vi "ADO Connection Create Table if Not Exist.vi"(6 "use file? (F)":bool, 7 "parameters":T1[](array[typedef]), 8 "error in (no error)":errorcluster caption="错误输入（无错误）", 9 "columns":string[](array[string]), 10 "table name":string, 11 "Database Connection 输入":refnum<class "Database Connection.lvclass"> caption="DNL_LabVIEW Object in") -> (0 "error out":errorcluster caption="错误输出", 1 "columns out":string[](array[string]), 2 "table":string, 3 "Database Connection 输出":refnum<class "Database Connection.lvclass"> caption="DNL_LabVIEW Object out")   [LabVIEW 2011, in "Database Connection.lvclass"]
uses:
  Database Connection.lvclass
  <vilib>/addons/database/Auxilliary.llb/DB Tools Parameter Info.ctl
  <vilib>/addons/database/Auxilliary.llb/DB Tools DataTypes.ctl
  <vilib>/addons/database/Auxilliary.llb/DB Tools Parameter Dir.ctl
  <vilib>/addons/database/NI_Database_API.lvlib
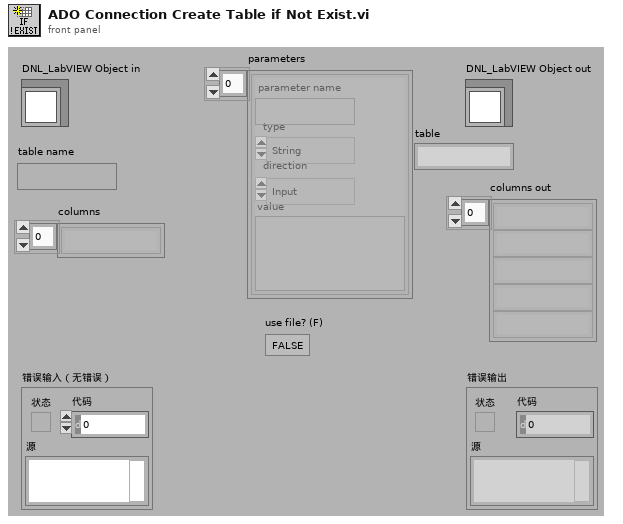
[diagram p1: front panel]
types:
  T1 = typedef "NI_Database_API.lvlib/DB Tools Parameter Info.ctl" = cluster{"parameter name":string, "type":T2, "direction":T3, "value":variant}
  T2 = typedef "NI_Database_API.lvlib/DB Tools DataTypes.ctl" = enum16{"String", "Long (I32)", "Single (SGL)", "Double (DBL)", "Date/Time", "Binary"}
  T3 = typedef "NI_Database_API.lvlib/DB Tools Parameter Dir.ctl" = enum32{"Input", "Output", "Input/Output", "Return Value"}
  T4 = cluster{"column name":string, "data type":T2, "size":i32, "allow null?":bool}
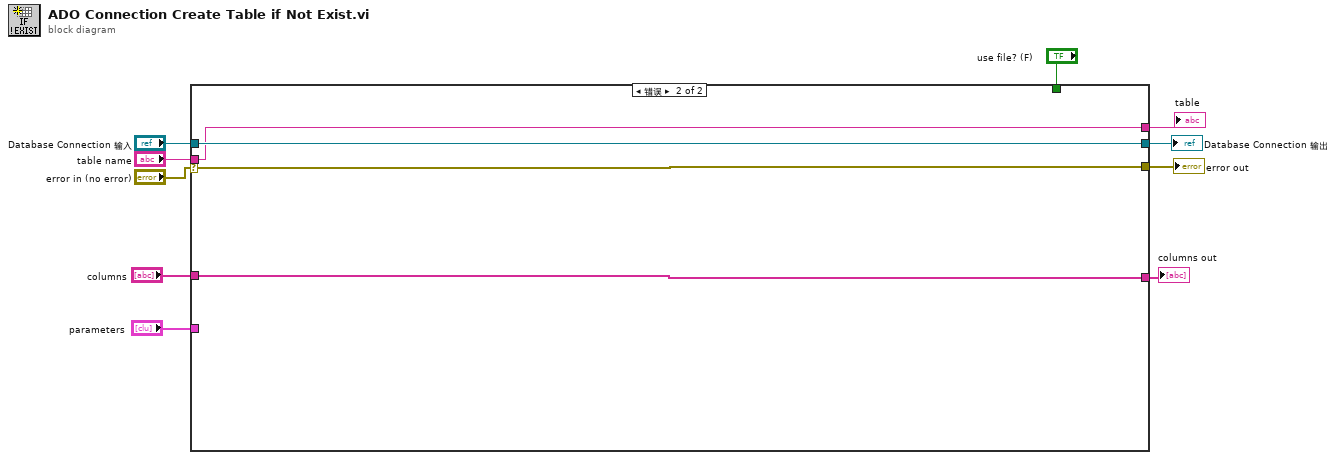
[diagram p0: block diagram]
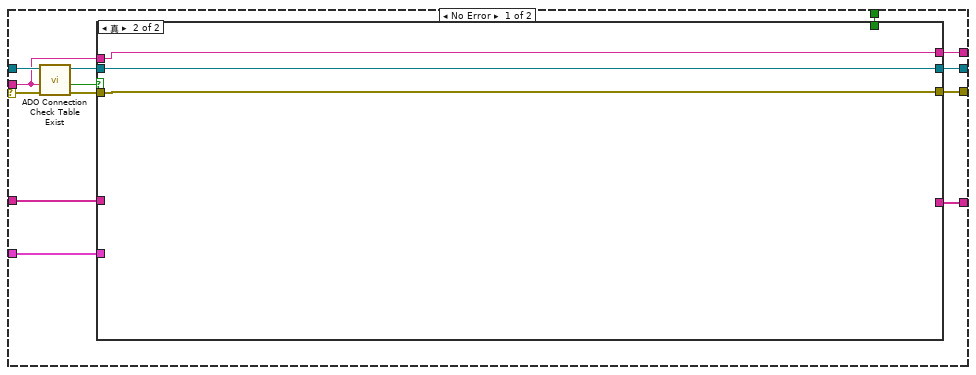
[diagram p2: hidden frame]
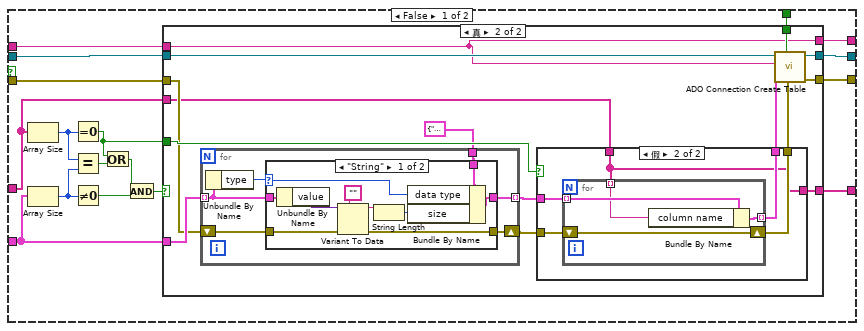
[diagram p3: hidden frame]
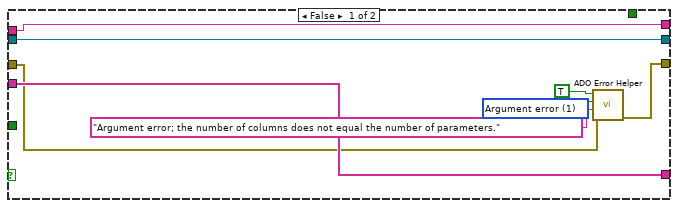
[diagram p4: hidden frame]
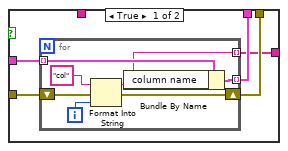
[diagram p5: hidden frame]
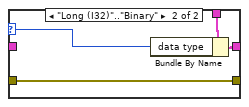
[diagram p6: hidden frame]
diagram:
  n1 = case shown="错误" "error in (no error)" {
    selector: "error in (no error)" -> [w22 w111]
    tunnel: [w17 w111] -> w9
    tunnel: [w19 w110] -> w7
    tunnel: "Database Connection 输入" -> [w23 w110]
    tunnel: "table name" -> [w12 w108]
    tunnel: "columns" -> [w16 w109]
    tunnel: "parameters" -> [w15 _]
    tunnel: [w14 w109] -> w3
    tunnel: "use file? (F)" -> [w13 _]
    tunnel: [w11 w108] -> w1
    frame No Error {
      n2 = call "ADO Connection Check Table Exist.vi"("error in (no error)"=w22, "table name"=w12, "Database Connection 输入"=w23) -> ("error out"=w18:errorcluster, "Exists?"=w21:bool, "Database Connection 输出"=w20:refnum<class "Database Connection.lvclass">)  [unwired: 6 in]
      n3 = case shown="真" w21 {
        tunnel: w20 -> [w33 w107]
        tunnel: [w31 w107] -> w19
        tunnel: w18 -> [w32 w106]
        tunnel: [w30 w106] -> w17
        tunnel: w16 -> [w29 _]
        tunnel: w15 -> [w34 _]
        tunnel: [w27 _] -> w14
        tunnel: w13 -> [w26 _]
        tunnel: w12 -> [w25 w105]
        tunnel: [w24 w105] -> w11
        frame False {
          n4 = Array Size(array=w29) -> (size(s)=w36:i32)
          n5 = Array Size(array=w34) -> (size(s)=w40:i32)
          n6 = Equal To 0?(x=w36) -> (x = 0?=w35:bool)
          n7 = Equal?(x=w36, y=w40) -> (x = y?=w37:bool)
          n8 = Not Equal To 0?(x=w40) -> (x != 0?=w39:bool)
          n9 = Or(x=w35, y=w37) -> (x .or. y?=w38:bool)
          n10 = And(x=w38, y=w39) -> (x .and. y?=w28:bool)
          n11 = case shown="真" w28 {
            tunnel: [w46 w63] -> w30
            tunnel: [w43 w62] -> w31
            tunnel: [w44 w57] -> w27
            tunnel: w35 -> [_ w56]
            tunnel: w34 -> [_ w55]
            tunnel: w33 -> [w43 w54]
            tunnel: w32 -> [w42 w53]
            tunnel: w29 -> [w44 w52]
            tunnel: w26 -> [_ w51]
            tunnel: w25 -> [w41 w49]
            tunnel: [w41 w49] -> w24
            frame False {
              w48 = 1 items=["No error", "Argument error", "Memory is full", "Out of zone", "End of file", "File already open", "Generic file I/O error", "File not found", "File permission error", "Disk is full", "Duplicate path", "Too many files open", "System feature not enabled", "Resource file not found", "Cannot add resource", "Resource not found", "Image not found", "Image memory error", "Pen does not exist", "Config type invalid", "Config token not found", "Config parse error", "Config memory error", "Bad external code format", "Bad external code offset", "External code not present", "Null window", "Destroy window error", "Null menu", "Print aborted", "Bad print record", "Print driver error", "Windows error during printing", "Memory error during printing", "Print dialog error", "Generic print error", "Invalid device refnum", "Device not found", "Device parameter error", "Device unit error", "Cannot open device", "Device call aborted", "Generic error", "Cancelled by user", "Object ID too low", "Object ID too high", "Object not in heap", "Unknown heap", "Unknown object (invalid DefProc)", "Unknown object (DefProc not in table)", "Message out of range", "Invalid (null) method", "Unknown message", "Manager call not supported", "Bad address", "Network operation in progress", "Network operation timed out", "Connection is busy", "Network attribute not supported", "Network error", "Address in use", "System out of memory", "Connection aborted", "Connection refused", "Not connected", "Already connected", "Connection closed", "Initialization error (interapplication manager)", "Bad occurrence", "Wait on unbound occurrence handler", "Occurrence queue overflow", "Datalog type conflict", "Unused", "Unrecognized type (interapplication manager)", "Memory corrupt", "Failed to make temporary DLL", "Old CIN version", "Drag socket not found", "Failed to load drop-object", "Failed to register OLE object", "Failed to release OLE object", "Format specifier type mismatch", "Unknown format specifier", "Too few format specifiers", "Too many format specifiers", "Scan failed", "Newer CIN version", "Error converting to variant", "Runtime menu error", "Password tampered", "Variant attribute not found", "Incompatible variant data type", "Event data is not available", "Event Store is not present", "Occurrence is not found", "Event Queue is not created", "Event info is not available", "Refnum passed is NULL", "Error retrieving Class GUID", "Error retrieving CoClass GUID", "Error retrieving TypeLib GUID.", "Bad built application magic bytes.", "Specific driver is different from the specific driver associated with the Logical Name.", "There is no session opened to the class driver.", "Max Error", "MAX - Error with config objects", "MAX - Error loading configuration", "MAX - Group not supported"]
              n12 = call "ADO Error Helper.vi"("Overriding error or warning"=w42, "source"="Argument error; the number of columns does not equal the number of parameters.", "code"=w48, "status"=TRUE) -> ("error out"=w46:errorcluster)  [unwired: 7 in]
            }
            frame True {
              n13 = for {
                shift-right: [w88] -> w58
                shift-left: w53 -> [w89]
                tunnel: T4 {"column name"="aa", "data type"=enum."String", "size"=0, "allow null?"=TRUE} ("column information") -> [w90]
                tunnel: [w87] -> w61 mode=indexing
                tunnel: w55 -> [w86] mode=indexing
                n14 = Unbundle By Name(w86) -> ("type"=w85:T2)
                n15 = case shown="\"String\"" w85 {
                  selector: w85 -> [w93 w101]
                  tunnel: [w97 w103] -> w87
                  tunnel: w90 -> [w94 w102]
                  tunnel: w89 -> [w96 w104]
                  tunnel: [w95 w104] -> w88
                  tunnel: w86 -> [w92 _]
                  frame "String" {
                    n16 = Unbundle By Name(w92) -> ("value"=w91:variant)
                    n17 = Variant To Data(error in=w96, type="", Variant=w91) -> (data=w99:string, error out=w95:errorcluster)
                    n18 = String Length(string=w99) -> (length=w98:i32)
                    n19 = Bundle By Name(cluster=w94, "data type"=w93, "size"=w98) -> (w97:T4)
                  }
                  frame "Long (I32)".."Binary" {
                    n20 = Bundle By Name(cluster=w102, "data type"=w101) -> (w103:T4)
                  }
                }
              }
              n21 = case shown="假" w56 {
                tunnel: w61 -> [w68 w80]
                tunnel: [w67 w79] -> w60
                tunnel: [w66 w78] -> w59
                tunnel: w58 -> [w65 w77]
                tunnel: [w64 w76] -> w57
                tunnel: w52 -> [_ w76]
                frame True {
                  n22 = for {
                    shift-right: [w73] -> w66
                    shift-left: w65 -> [w74]
                    tunnel: [w72] -> w67 mode=indexing
                    tunnel: w68 -> [w71] mode=indexing
                    tunnel: [w69] -> w64 mode=indexing
                    i -> [w75]
                    n23 = Format Into String(initial string="col", error in=w74, w75) -> (resulting string=w69:string, error out=w73:errorcluster)  [unwired: 1 in]
                    n24 = Bundle By Name(cluster=w71, "column name"=w69) -> (w72:T4)
                  }
                }
                frame False {
                  n25 = for {
                    shift-right: [w82] -> w78
                    shift-left: w77 -> [w82]
                    tunnel: [w84] -> w79 mode=indexing
                    tunnel: w80 -> [w83] mode=indexing
                    tunnel: w76 -> [w81] mode=indexing
                    n26 = Bundle By Name(cluster=w83, "column name"=w81) -> (w84:T4)
                  }
                }
              }
              n27 = call "ADO Connection Create Table.vi"("file?"=w51, "error in (no error)"=w59, "column information"=w60, "table"=w49, "Database Connection.lvclass In"=w54) -> ("error IO"=w63:errorcluster, "Database Connection.lvclass Out"=w62:refnum<class "Database Connection.lvclass">)  [unwired: 5 in]
            }
          }
        }
        frame True {
        }
      }
    }
    frame Error {
    }
  }
  "error out" <- w9
  "Database Connection 输出" <- w7
  "columns out" <- w3
  "table" <- w1
